vi "Save Data (SubVI).vi"(0 "Save Enable":bool, 5 "Save Interval [sec]":dbl=1.0 min=0.0 step=0.1, 7 "File Name":string, 9 "Folder Location":path, 11 "Data Array (Row)":string[](array[string]), 12 "Column Header Array":string[](array[string]), 13 "Title Block":string[][](array[string]), 14 "External Save Signal":bool) -> (4 "File Path":path, 8 "Row Count":u16, 15 "Save Error":errorcluster)   [LabVIEW 2012]
panel:
  # "SAVE DATA\nCreated by Blake Otting \nLast Update 3-6-2013"
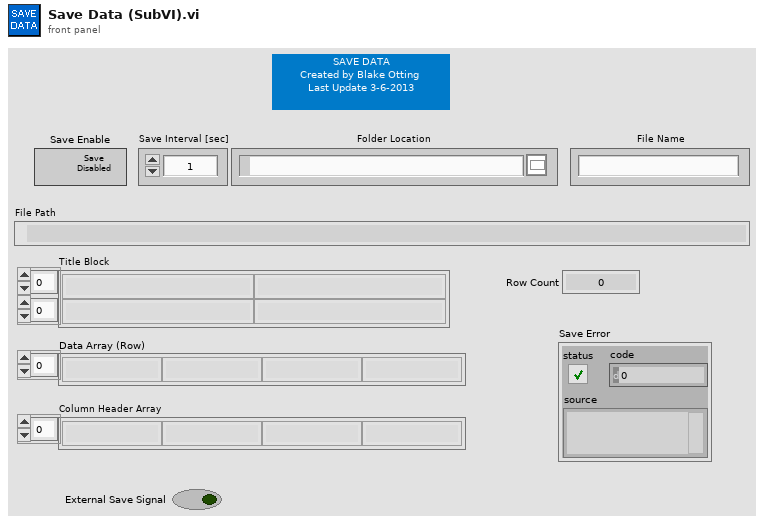
[diagram p1: front panel]
types:
  T1 = enum16{"open", "replace", "create", "open or create", "replace or create", "replace or create with confirmation"}
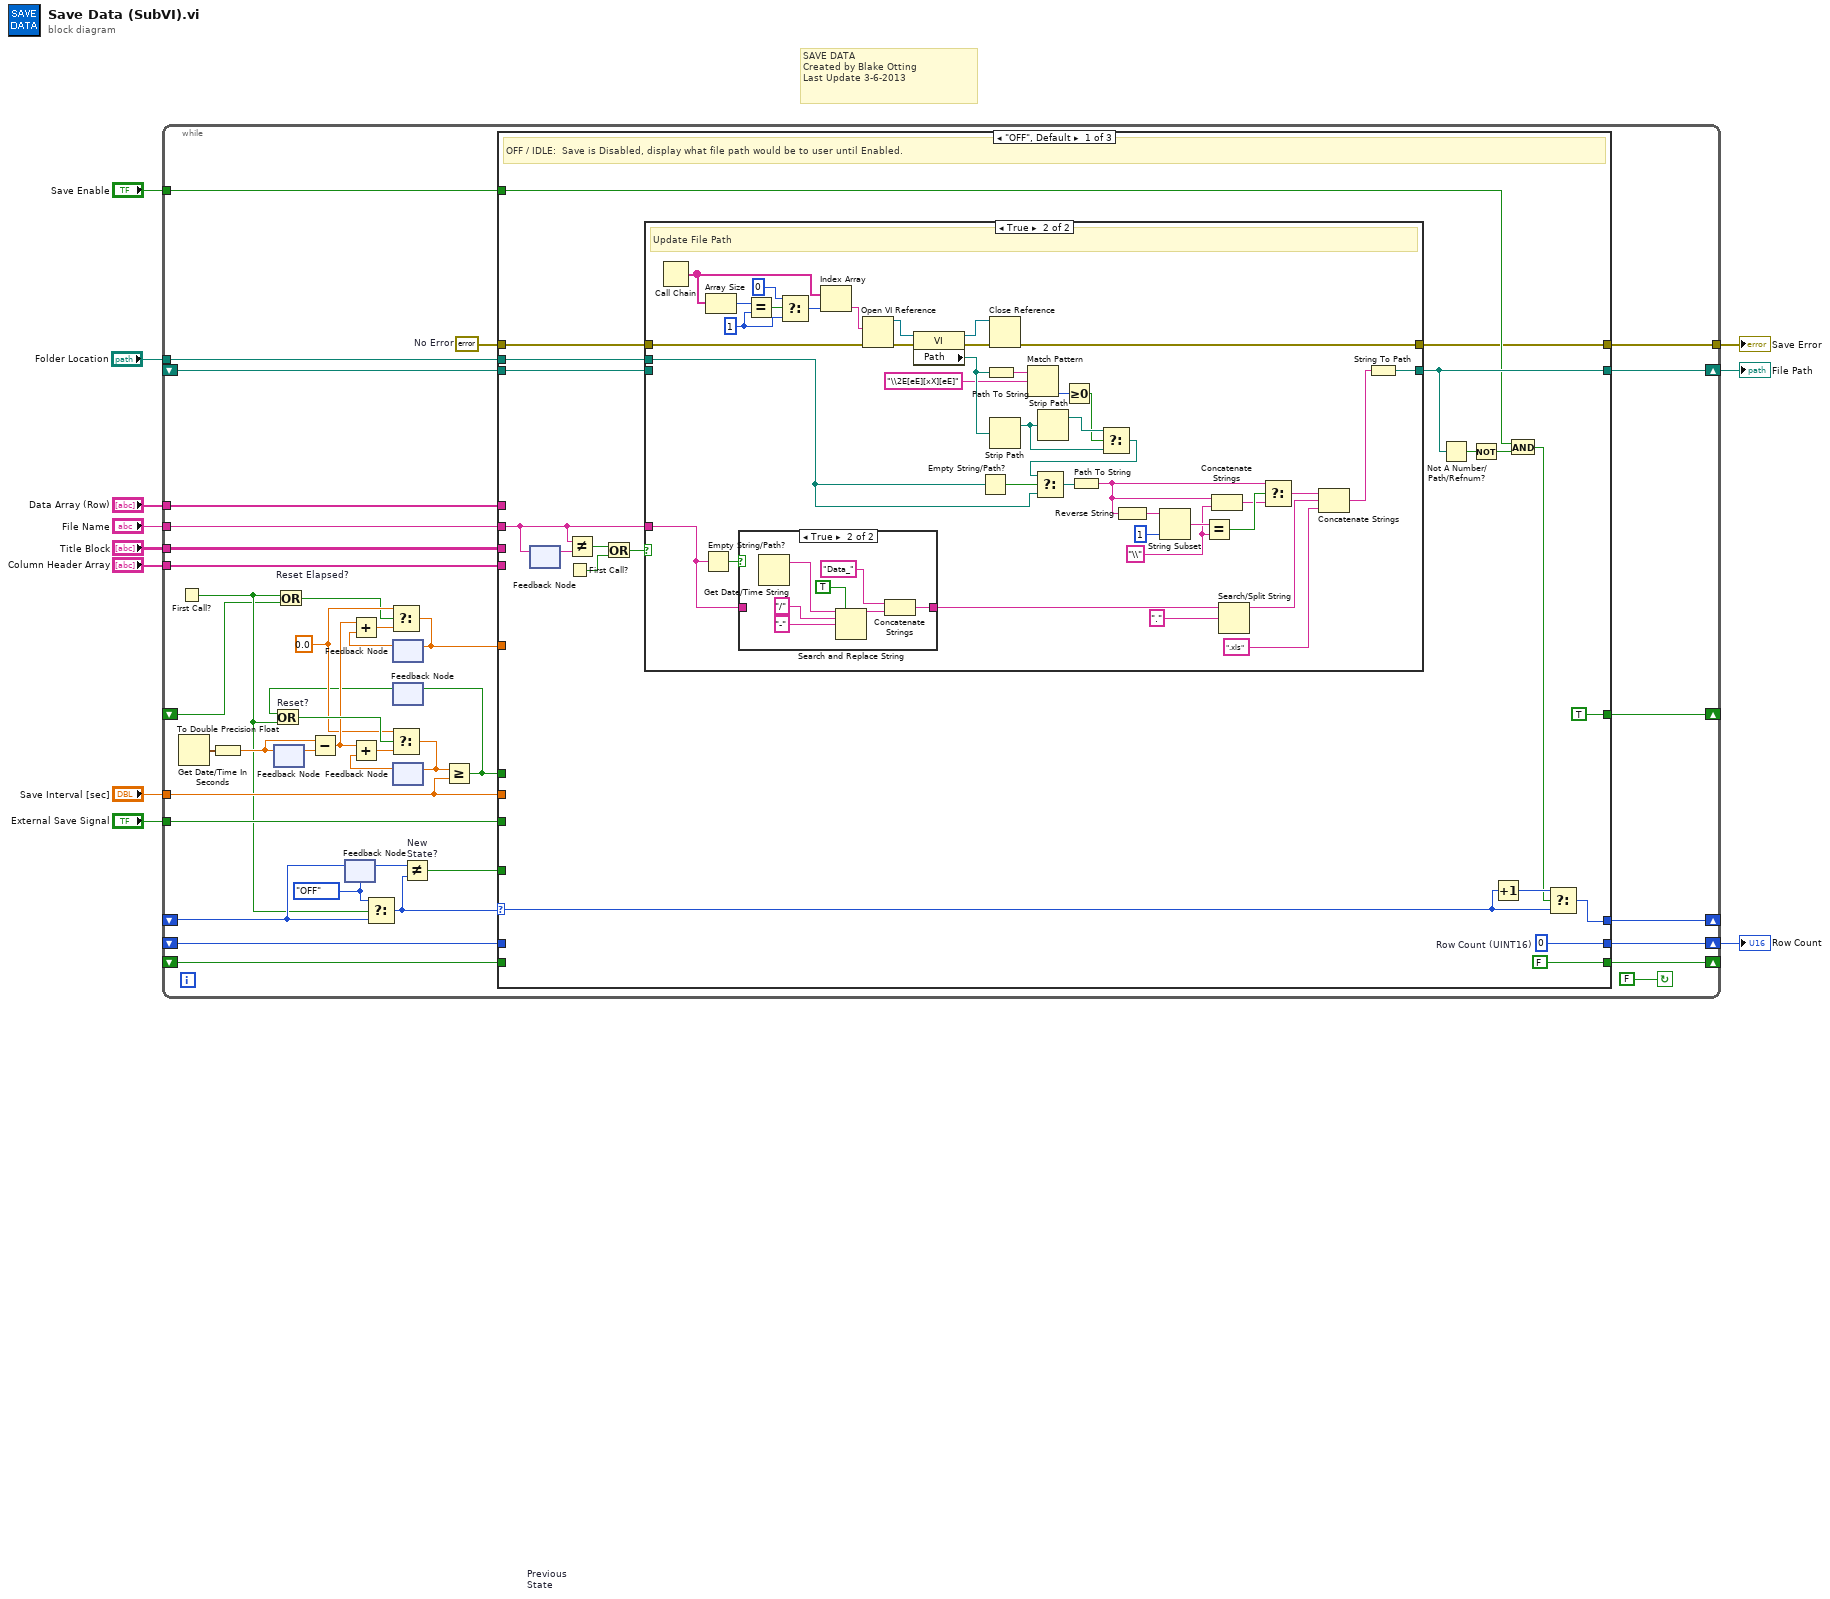
[diagram p0: block diagram]
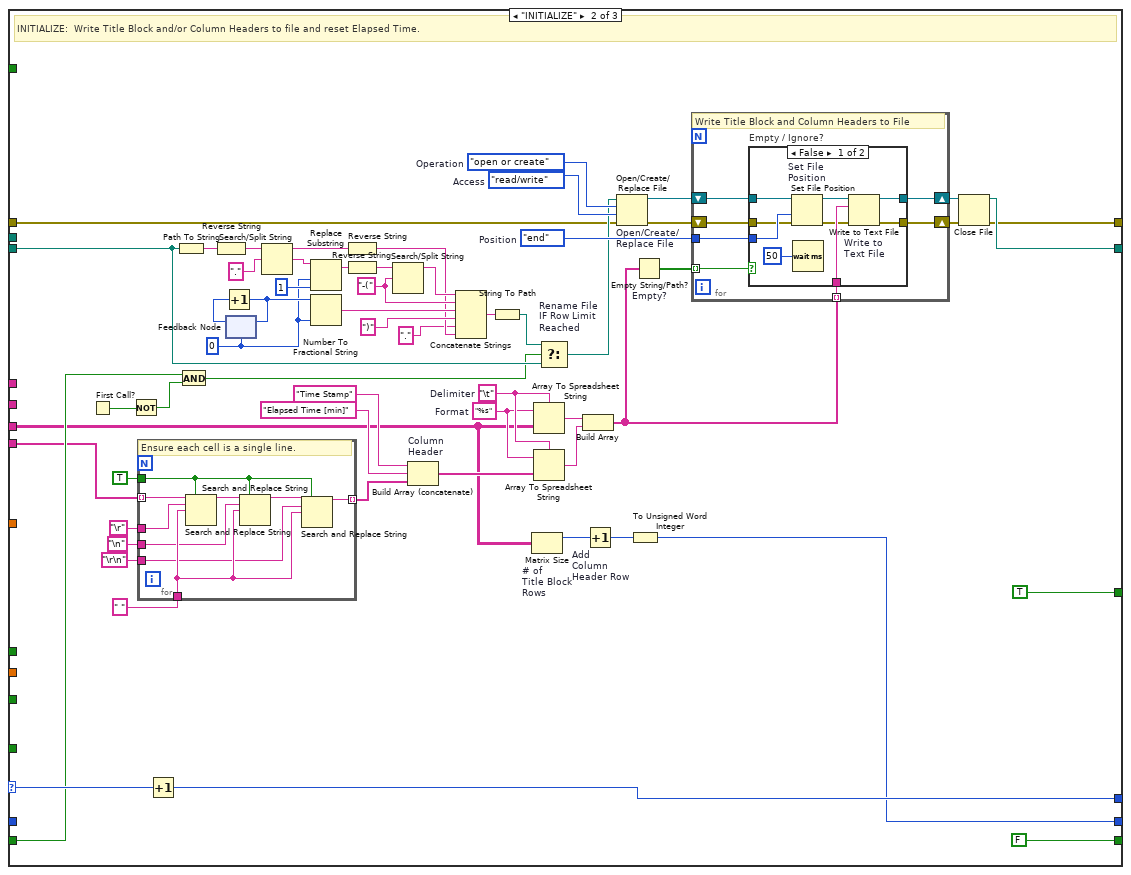
[diagram p4: hidden frame]
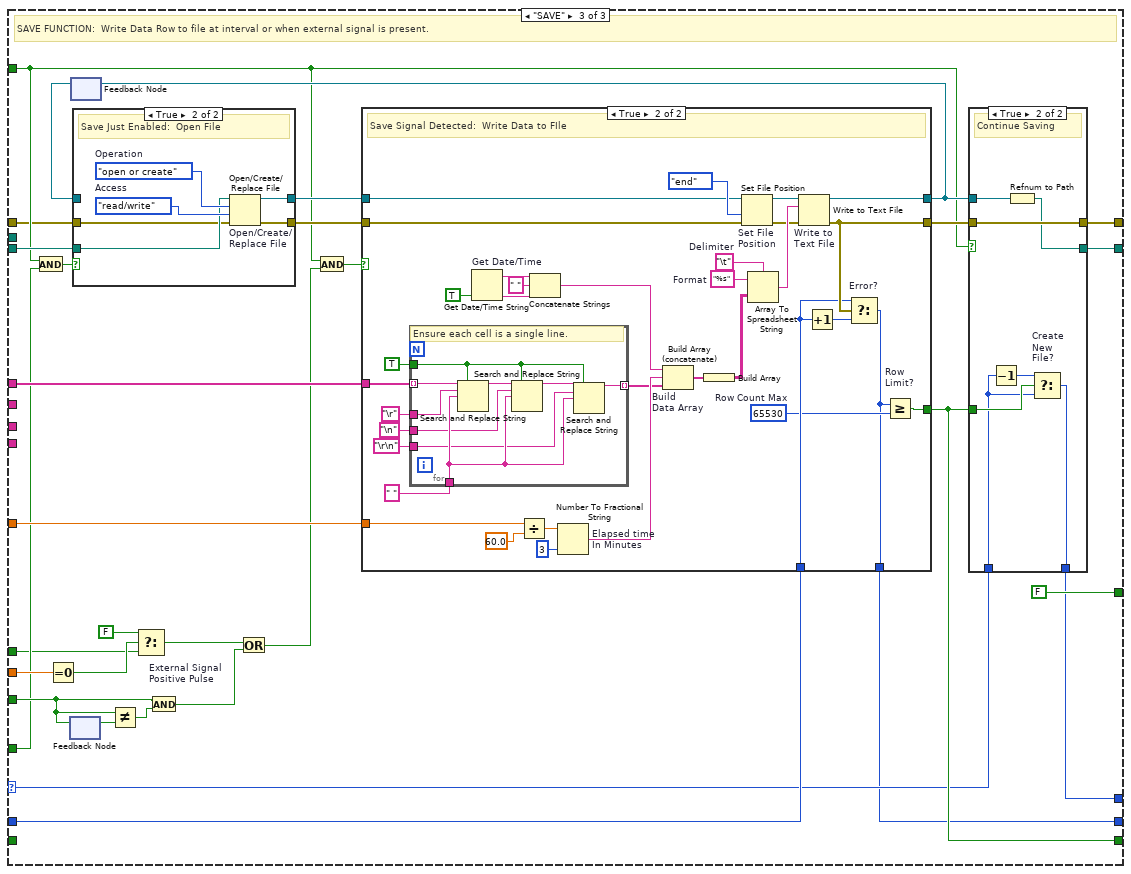
[diagram p6: hidden frame]
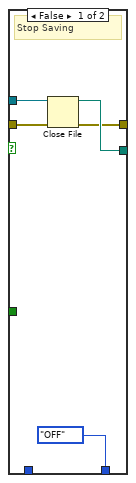
[diagram p8: hidden frame]
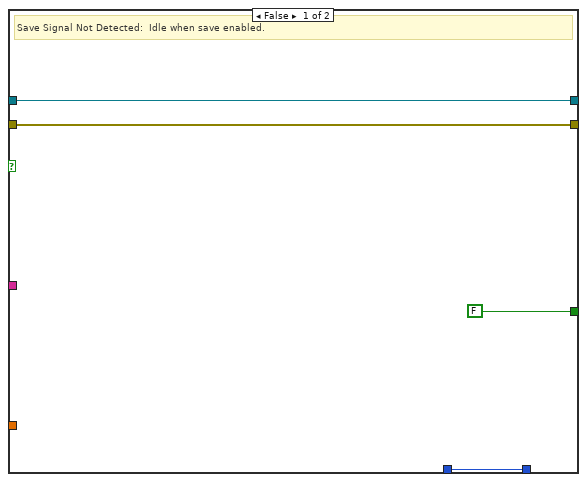
[diagram p9: hidden frame]
diagram:
  # "SAVE DATA\nCreated by Blake Otting \nLast Update 3-6-2013"
  n1 = while {
    tunnel: "Save Enable" -> [w24]
    shift-right: [w51] -> _
    shift-left: _ -> [w26]
    shift-right: [w50] -> w2
    shift-left: _ -> [w49]
    tunnel: "Title Block" -> [w48]
    tunnel: "Column Header Array" -> [w47]
    tunnel: "Data Array (Row)" -> [w46]
    shift-right: [w45] -> w3
    shift-left: _ -> [w44]
    shift-right: [w43] -> _
    shift-left: _ -> [w42]
    shift-right: [w30] -> _
    shift-left: _ -> [w14]
    tunnel: "Save Interval [sec]" -> [w18]
    tunnel: "Folder Location" -> [w29]
    tunnel: "File Name" -> [w28]
    tunnel: "External Save Signal" -> [w23]
    tunnel: [w27] -> w1
    stop <- FALSE continue-if-true
    w12 = errorcluster {"status"=FALSE, "code"=0, "source"=""}  # No Error
    w31 = 0.0 ("t")
    w25 = enum16{"OFF", "INITIALIZE", "SAVE"}."OFF"
    n2 = First Call?() -> (First Call?: T/F=w15:bool)
    n3 = Get Date/Time In Seconds() -> (seconds since 1Jan1904=w39:timestamp)
    n4 = To Double Precision Float(number=w39) -> (double precision float=w35:dbl)
    n5 = feedback #1() -> (w40:dbl)  [unwired: 1 in]
    n6 = feedback-in #1(w35) -> ()
    n7 = Or "Reset Elapsed?"(x=w15, y=w14) -> (x .or. y?=w13:bool)
    n8 = Subtract(x=w35, y=w40) -> (x-y=w32:dbl)
    n9 = feedback-in #2(w26) -> ()
    n10 = feedback #2 "Previous\nState"(w25) -> (w22:enum16{"OFF", "INITIALIZE", "SAVE"})
    n11 = Select(t=w25, s=w15, f=w26) -> (s? t:f=w21:enum16{"OFF", "INITIALIZE", "SAVE"})
    n12 = feedback #3() -> (w33:dbl)  [unwired: 1 in]
    n13 = Add(x=w32, y=w33) -> (x+y=w36:dbl)
    n14 = Select(t=w31, s=w13, f=w36) -> (s? t:f=w41:dbl)
    n15 = feedback-in #3(w41) -> ()
    n16 = feedback #4() -> (w16:bool)  [unwired: 1 in]
    n17 = Or "Reset?"(x=w16, y=w15) -> (x .or. y?=w37:bool)
    n18 = feedback #5() -> (w34:dbl)  [unwired: 1 in]
    n19 = Add(x=w32, y=w34) -> (x+y=w38:dbl)
    n20 = Select(t=w31, s=w37, f=w38) -> (s? t:f=w19:dbl)
    n21 = feedback-in #5(w19) -> ()
    n22 = Not Equal? "New\nState?"(x=w22, y=w21) -> (x != y?=w20:bool)
    n23 = Greater Or Equal?(x=w19, y=w18) -> (x >= y?=w17:bool)
    n24 = feedback-in #4(w17) -> ()
    n25 = case shown="\"OFF\", Default" w21 {
      selector: w21 -> [w71 w181 w212]
      tunnel: [w70 w180 w211] -> w51
      tunnel: w24 -> [w57 _ w217]
      tunnel: [w69 w170 w210] -> w50
      tunnel: w49 -> [_ _ w228]
      tunnel: w48 -> [_ w135 _]
      tunnel: w44 -> [w53 w169 w232]
      tunnel: w47 -> [_ w125 _]
      tunnel: w46 -> [_ _ w238]
      tunnel: w41 -> [_ _ w239]
      tunnel: [w58 w132 w234] -> w45
      tunnel: [FALSE FALSE w213] -> w43
      tunnel: w42 -> [_ w165 _]
      tunnel: [TRUE TRUE FALSE] -> w30
      tunnel: w29 -> [w67 _ _]
      tunnel: w28 -> [w64 _ _]
      tunnel: w18 -> [_ _ w220]
      tunnel: w23 -> [_ _ w219]
      tunnel: [w54 w131 w235] -> w27
      tunnel: w20 -> [_ _ w218]
      tunnel: w17 -> [_ _ w214]
      tunnel: w12 -> [w55 w123 w209]
      frame "OFF", Default {
        w69 = u16 0  # Row Count (UINT16)
        # "OFF / IDLE:  Save is Disabled, display what file path would be to user until Enabled."
        n26 = feedback-in #6(w64) -> ()
        n27 = feedback #6() -> (w63:string)  [unwired: 1 in]
        n28 = First Call?() -> (First Call?: T/F=w65:bool)
        n29 = Not Equal?(x=w64, y=w63) -> (x != y?=w62:bool)
        n30 = Or(x=w62, y=w65) -> (x .or. y?=w61:bool)
        n31 = case shown="True" w61 {
          tunnel: w67 -> [_ w100]
          tunnel: [w73 w99] -> w58
          tunnel: w64 -> [_ w78]
          tunnel: w55 -> [w74 w76]
          tunnel: [w74 w75] -> w54
          tunnel: w53 -> [w73 _]
          frame False {
            # "File Path hasn't changed, do nothing."
          }
          frame True {
            w86 = 1 ("index")
            w106 = "\\"
            # "Update File Path"
            n32 = Call Chain() -> (call chain=w82:string[])
            n33 = Empty String/Path?(string/path=w78) -> (empty?=w98:bool)
            n34 = Array Size(array=w82) -> (size(s)=w85:i32)
            n35 = case shown="True" w98 {
              tunnel: w78 -> [w115 _]
              tunnel: [w115 w116] -> w97
              frame False {
              }
              frame True {
                n36 = Get Date/Time String() -> (date string=w120:string)  [unwired: 3 in, 1 out]
                n37 = Search and Replace String(replace all?=TRUE, input string=w120, search string="/", replace string="-") -> (result string=w117:string)  [unwired: 4 in, 3 out]
                n38 = Concatenate Strings("Data_" ("search string/char (-)"), w117) -> (w116:string)
              }
            }
            n39 = Equal?(x=w85, y=w86) -> (x = y?=w83:bool)
            n40 = Select(t=0, s=w83, f=w86) -> (s? t:f=w84:i32)
            n41 = Index Array(array=w82, index=w84) -> (element=w90:string)
            n42 = Open VI Reference(vi path=w90, error in (no error)=w76) -> (vi reference=w89:refnum<vi>, error out=w88:errorcluster)  [unwired: 4 in]
            n43 = property class="VI"(reference=w89, error in=w88) -> (reference out=w92:refnum<vi>, error out=w91:errorcluster, "Path"=w94:path)
            n44 = Empty String/Path?(string/path=w100) -> (empty?=w103:bool)
            n45 = Path To String(path=w94) -> (string=w80:string)
            n46 = Close Reference(reference=w92, error in (no error)=w91) -> (error out=w75:errorcluster)
            n47 = Strip Path(path=w94) -> (stripped path=w95:path)  [unwired: 1 out]
            n48 = Match Pattern(string=w80, regular expression="\\2E[eE][xX][eE]") -> (offset past match=w79:i32)  [unwired: 1 in, 3 out]
            n49 = Strip Path(path=w95) -> (stripped path=w96:path)  [unwired: 1 out]
            n50 = Greater Or Equal To 0?(x=w79) -> (x >= 0?=w93:bool)
            n51 = Select(t=w96, s=w93, f=w95) -> (s? t:f=w77:path)
            n52 = Select(t=w77, s=w103, f=w100) -> (s? t:f=w102:path)
            n53 = Path To String(path=w102) -> (string=w101:string)
            n54 = Reverse String(1:w101) -> (0:w110:string)
            n55 = String Subset(string=w110, length (rest)=1) -> (substring=w108:string)  [unwired: 1 in]
            n56 = Equal?(x=w108, y=w106) -> (x = y?=w107:bool)
            n57 = Concatenate Strings(w101, w106) -> (w105:string)
            n58 = Search/Split String(string=w97, search string/char (-)=".") -> (substring before match=w111:string)  [unwired: 1 in, 2 out]
            n59 = Select(t=w101, s=w107, f=w105) -> (s? t:f=w104:string)
            n60 = Concatenate Strings(w104, w111, ".xls" ("string")) -> (w113:string)
            n61 = String To Path(string=w113) -> (path=w99:path)
          }
        }
        n62 = Not A Number/Path/Refnum?(number/path/refnum=w58) -> (NaN/Path/Refnum?=w59:bool)
        n63 = Not(x=w59) -> (.not. x?=w60:bool)
        n64 = Increment(x=w71) -> (x+1=w72:enum16{"OFF", "INITIALIZE", "SAVE"})
        n65 = And(x=w57, y=w60) -> (x .and. y?=w56:bool)
        n66 = Select(t=w72, s=w56, f=w71) -> (s? t:f=w70:enum16{"OFF", "INITIALIZE", "SAVE"})
      }
      frame "INITIALIZE" {
        w142 = enum16{"read/write", "read-only", "write-only"}."read/write"  # Access
        w146 = u8 0
        w154 = "-("
        w173 = enum16{"start", "end", "current"}."end"  # Position
        w143 = T1."open or create"  # Operation
        w179 = "\t"  # Delimiter
        w178 = "%s"  # Format
        # "INITIALIZE:  Write Title Block and/or Column Headers to file and reset Elapsed Time."
        n67 = First Call?() -> (First Call?: T/F=w164:bool)
        n68 = Not(x=w164) -> (.not. x?=w167:bool)
        n69 = for {
          tunnel: w125 -> [w190] mode=indexing
          tunnel: TRUE -> [w188]
          tunnel: [w186] -> w124 mode=indexing
          tunnel: " " ("replace string (\"\")") -> [w185]
          tunnel: "\r" -> [w184]
          tunnel: "\n" -> [w183]
          tunnel: "\r\n" -> [w182]
          # "Ensure each cell is a single line."
          n70 = Search and Replace String(replace all?=w188, input string=w190, search string=w184, replace string=w185) -> (result string=w189:string)  [unwired: 4 in, 3 out]
          n71 = Search and Replace String(replace all?=w188, input string=w189, search string=w183, replace string=w185) -> (result string=w187:string)  [unwired: 4 in, 3 out]
          n72 = Search and Replace String(replace all?=w188, input string=w187, search string=w182, replace string=w185) -> (result string=w186:string)  [unwired: 4 in, 3 out]
        }
        n73 = Increment(x=w181) -> (x+1=w180:enum16{"OFF", "INITIALIZE", "SAVE"})
        n74 = Path To String(path=w169) -> (string=w157:string)
        n75 = And(x=w165, y=w167) -> (x .and. y?=w166:bool)
        n76 = Reverse String(1:w157) -> (0:w158:string)
        n77 = feedback #7(w146) -> (w152:u8)
        n78 = Increment(x=w152) -> (x+1=w153:u8)
        n79 = feedback-in #7(w153) -> ()
        n80 = Search/Split String(string=w158, search string/char (-)=".") -> (substring before match=w159:string, match + rest of string=w160:string)  [unwired: 2 out]
        n81 = Replace Substring(2:1 ("length (len. of substring)"), 3:w146, 5:w160) -> (1:w161:string)  [unwired: 2 out]
        n82 = Number To Fractional String(number=w153, precision (6)=w146) -> (F-format string=w163:string)  [unwired: 2 in]
        n83 = Reverse String(1:w159) -> (0:w149:string)
        n84 = Reverse String(1:w161) -> (0:w155:string)
        n85 = Search/Split String(string=w155, search string/char (-)=w154) -> (substring before match=w151:string)  [unwired: 1 in, 2 out]
        n86 = Build Array (concatenate) "Column\nHeader"("Time Stamp", "Elapsed Time [min]", w124) -> (w176:string[])
        n87 = Concatenate Strings(w151, w154, w163, ")", "." ("search string/char (-)"), w149) -> (w148:string)
        n88 = String To Path(string=w148) -> (path=w168:path)
        n89 = Matrix Size "# of\nTitle Block\nRows"(0:w135) -> (1:w172:i32)  [unwired: 1 out]
        n90 = Array To Spreadsheet String(delimiter (Tab)=w179, array=w135, 3:w178) -> (spreadsheet string=w175:string)
        n91 = Array To Spreadsheet String(delimiter (Tab)=w179, array=w176, 3:w178) -> (spreadsheet string=w174:string)
        n92 = Select "Rename File\nIF Row Limit\nReached"(t=w168, s=w166, f=w169) -> (s? t:f=w137:path)
        n93 = Build Array(w175, w174) -> (w139:string[])
        n94 = Increment "Add\nColumn\nHeader Row"(x=w172) -> (x+1=w171:i32)
        n95 = Open/Create/Replace File "Open/Create/\nReplace File"(file path (use dialog)=w137, error in=w123, operation (0:open)=w143, access (0:read/write)=w142) -> (refnum out=w141:refnum<file>, error out=w140:errorcluster)  [unwired: 2 in, 1 out]
        n96 = To Unsigned Word Integer(number=w171) -> (unsigned 16bit integer=w170:u16)
        n97 = Empty String/Path? "Empty?"(string/path=w139) -> (empty?=w138:bool[])
        n98 = for {
          tunnel: w139 -> [w196] mode=indexing
          tunnel: w173 -> [w195]
          shift-right: [w197] -> w133
          shift-left: w140 -> [w194]
          shift-right: [w192] -> w134
          shift-left: w141 -> [w193]
          tunnel: w138 -> [w191] mode=indexing
          # "Write Title Block and Column Headers to File"
          n99 = case "Empty / Ignore?" shown="False" w191 {
            tunnel: [w205 w208] -> w197
            tunnel: [w204 w207] -> w192
            tunnel: w196 -> [w203 _]
            tunnel: w195 -> [w202 _]
            tunnel: w194 -> [w201 w208]
            tunnel: w193 -> [w200 w207]
            frame False {
              n100 = Set File Position "Set File \nPosition"(refnum=w200, from (0:start)=w202, error in=w201) -> (refnum out=w198:refnum<file>, error out=w199:errorcluster)  [unwired: 1 in]
              n101 = Wait (ms)(milliseconds to wait=u32 50) -> ()  [unwired: 1 out]
              n102 = Write to Text File "Write to \nText File"(file (use dialog)=w198, text=w203, error in=w199) -> (refnum out=w204:refnum<file>, error out=w205:errorcluster)  [unwired: 1 in, 1 out]
            }
            frame True {
            }
          }
        }
        n103 = Close File(refnum=w134, error in=w133) -> (path=w132:path, error out=w131:errorcluster)
      }
      frame "SAVE" {
        # "SAVE FUNCTION:  Write Data Row to file at interval or when external signal is present."
        n104 = And(x=w217, y=w218) -> (x .and. y?=w221:bool)
        n105 = Equal To 0?(x=w220) -> (x = 0?=w225:bool)
        n106 = feedback-in #8(w219) -> ()
        n107 = feedback #8() -> (w224:bool)  [unwired: 1 in]
        n108 = feedback #9() -> (w230:refnum<file>)  [unwired: 1 in]
        n109 = case shown="True" w221 {
          tunnel: w232 -> [_ w243]
          tunnel: [w240 w245] -> w231
          tunnel: w230 -> [w241 _]
          tunnel: [w241 w244] -> w229
          tunnel: w209 -> [w240 w242]
          frame False {
            # "File Previously Opened:  Use Ref"
          }
          frame True {
            w246 = enum16{"read/write", "read-only", "write-only"}."read/write"  # Access
            w247 = T1."open or create"  # Operation
            # "Save Just Enabled:  Open File"
            n110 = Open/Create/Replace File "Open/Create/\nReplace File"(file path (use dialog)=w243, error in=w242, operation (0:open)=w247, access (0:read/write)=w246) -> (refnum out=w244:refnum<file>, error out=w245:errorcluster)  [unwired: 2 in, 1 out]
          }
        }
        n111 = Not Equal?(x=w219, y=w224) -> (x != y?=w223:bool)
        n112 = Select(t=FALSE, s=w225, f=w214) -> (s? t:f=w226:bool)
        n113 = And "External Signal\nPositive Pulse"(x=w219, y=w223) -> (x .and. y?=w222:bool)
        n114 = Or(x=w226, y=w222) -> (x .or. y?=w216:bool)
        n115 = And(x=w217, y=w216) -> (x .and. y?=w215:bool)
        n116 = case shown="True" w215 {
          tunnel: w239 -> [_ w278]
          tunnel: w238 -> [_ w271]
          tunnel: w231 -> [w263 w284]
          tunnel: [w263 w269] -> w236
          tunnel: w229 -> [w262 w283]
          tunnel: [w262 w280] -> w233
          tunnel: w228 -> [w261 w267]
          tunnel: [w261 w265] -> w210
          tunnel: [FALSE w264] -> w213
          frame False {
            # "Save Signal Not Detected:  Idle when save enabled."
          }
          frame True {
            w266 = u16 65530  # Row Count Max
            w286 = "\t"  # Delimiter
            w289 = "%s"  # Format
            # "Save Signal Detected:  Write Data to FIle"
            n117 = for {
              tunnel: w271 -> [w306] mode=indexing
              tunnel: TRUE -> [w304]
              tunnel: [w302] -> w270 mode=indexing
              tunnel: " " ("replace string (\"\")") -> [w301]
              tunnel: "\r" -> [w300]
              tunnel: "\n" -> [w299]
              tunnel: "\r\n" -> [w298]
              # "Ensure each cell is a single line."
              n118 = Search and Replace String(replace all?=w304, input string=w306, search string=w300, replace string=w301) -> (result string=w305:string)  [unwired: 4 in, 3 out]
              n119 = Search and Replace String(replace all?=w304, input string=w305, search string=w299, replace string=w301) -> (result string=w303:string)  [unwired: 4 in, 3 out]
              n120 = Search and Replace String(replace all?=w304, input string=w303, search string=w298, replace string=w301) -> (result string=w302:string)  [unwired: 4 in, 3 out]
            }
            n121 = Get Date/Time String "Get Date/Time"(want seconds? (F)=TRUE) -> (date string=w290:string, time string=w293:string)  [unwired: 2 out]
            n122 = Divide(x=w278, y=60.0) -> (x/y=w277:dbl)
            n123 = Concatenate Strings(w290, " " ("string"), w293) -> (w294:string)
            n124 = Number To Fractional String "Elapsed time\nIn Minutes"(number=w277, precision (6)=i16 3) -> (F-format string=w287:string)  [unwired: 2 in]
            n125 = Build Array (concatenate) "Build\nData Array"(w294, w287, w270) -> (w295:string[])
            n126 = Build Array(w295) -> (w296:string[][])
            n127 = Set File Position "Set File \nPosition"(refnum=w283, from (0:start)=enum16{"start", "end", "current"}."end", error in=w284) -> (refnum out=w281:refnum<file>, error out=w282:errorcluster)  [unwired: 1 in]
            n128 = Array To Spreadsheet String(delimiter (Tab)=w286, array=w296, 3:w289) -> (spreadsheet string=w285:string)
            n129 = Write to Text File "Write to \nText File"(file (use dialog)=w281, text=w285, error in=w282) -> (refnum out=w280:refnum<file>, error out=w269:errorcluster)  [unwired: 1 in, 1 out]
            n130 = Increment(x=w267) -> (x+1=w268:u16)
            n131 = Select "Error?"(t=w267, s=w269, f=w268) -> (s? t:f=w265:u16)
            n132 = Greater Or Equal? "Row\nLimit?"(x=w265, y=w266) -> (x >= y?=w264:bool)
          }
        }
        n133 = feedback-in #9(w233) -> ()
        n134 = case shown="True" w217 {
          tunnel: w233 -> [w250 w258]
          tunnel: w236 -> [w252 w259]
          tunnel: [w249 w259] -> w235
          tunnel: [w251 w257] -> w234
          tunnel: w213 -> [_ w255]
          tunnel: w212 -> [_ w254]
          tunnel: [enum16{"OFF", "INITIALIZE", "SAVE"}."OFF" w253] -> w211
          frame False {
            # "Stop Saving"
            n135 = Close File(refnum=w250, error in=w252) -> (path=w251:path, error out=w249:errorcluster)
          }
          frame True {
            # "Continue Saving"
            n136 = Decrement(x=w254) -> (x-1=w256:enum16{"OFF", "INITIALIZE", "SAVE"})
            n137 = Refnum to Path(1:w258) -> (0:w257:path)
            n138 = Select "Create\nNew\nFile?"(t=w256, s=w255, f=w254) -> (s? t:f=w253:enum16{"OFF", "INITIALIZE", "SAVE"})
          }
        }
      }
    }
  }
  "File Path" <- w3
  "Row Count" <- w2
  "Save Error" <- w1
